vi "Lockin.vi"(4 "stop?":bool, 6 "initialize?":bool, 8 "error in (no error)":errorcluster, 11 "Transport":refnum<class "Transport.lvclass">) -> (0 "error out":errorcluster, 3 "Transport out":refnum<class "Transport.lvclass">)   [LabVIEW 2016, in "Transport.lvclass"]
uses:
  Transport.lvclass
  Control Experiment/Typedefs/Instruments--cluster.ctl
  <userlib>/LevyLab/Krohn Hite 7008/Instrument.KH7008.lvclass
  <userlib>/LevyLab/Lockin-Multichannel/Instrument.Lockin/Instrument.Lockin.lvclass
  <userlib>/LevyLab/Levylab Instruments/Instrument Types/Cryostat/Instrument.Cryostat.lvclass
  <userlib>/LevyLab/Levylab Instruments/Instrument Types/CBridge/Instrument.CBridge.lvclass
  <userlib>/LevyLab/Levylab Instruments/Instrument Types/Optical Delay Line/Instrument.OpticalDelayLine.lvclass
  <userlib>/LevyLab/Levylab Instruments/Instrument Types/Strain/Instrument.Strain.lvclass
  <userlib>/LevyLab/Levylab Instruments/Instrument Types/VNA/Instrument.VNA.lvclass
  <userlib>/LevyLab/Levylab Instruments/Instrument Types/VSource/Instrument.VSource.lvclass
  Transport.lvclass/Transport.ctl
  Control Experiment/Control Experiment.lvclass/Control Experiment.ctl
  SweepControl/SweepControl.lvclass/SweepControl.ctl
  Control Experiment/Control Experiment.lvclass
  SweepControl/SweepControl.lvclass
panel:
  in  "Tab Control":enum32{"lockin/SG Control", "Data", "Other"}(tab)
  out "elapsed time (s)":u32=76
  in  "Experiment Comments":string="describe only the experiment you're doing right now"
  in  "Experiment Folder":string="Experiment folder"
  out "T (mK)":dbl
  out "Field (T)":dbl=0.5 format="%#_13g"
  out "time b/w points (ms)":u32=76
  in  "stop":bool
  out "X Lockins":cluster{dbl[], dbl[]}[](graph)
  out "Y Lockins":cluster{dbl[], dbl[]}[](graph)
  out "G4T":cluster{dbl[], dbl[]}[](graph)
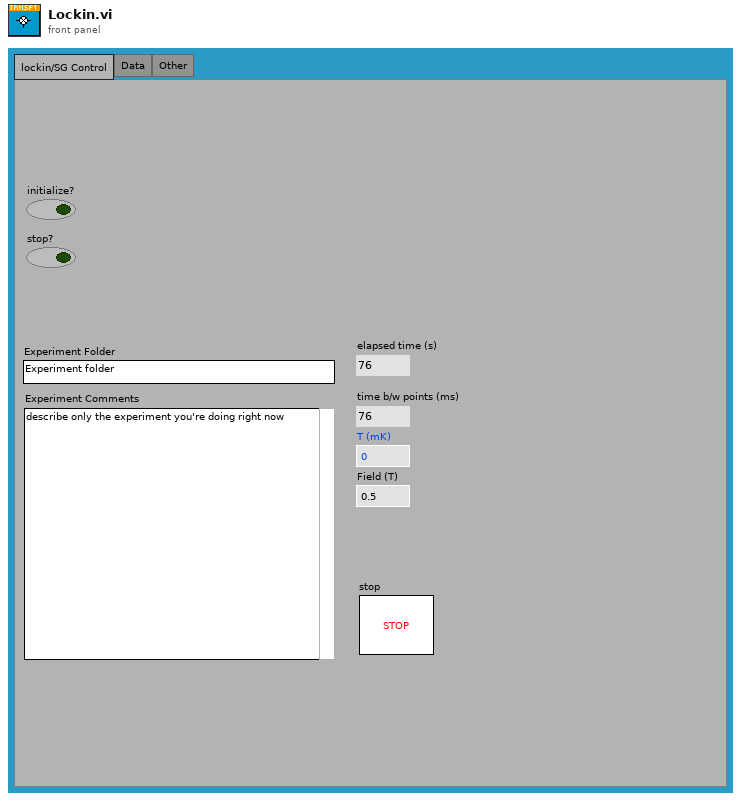
[diagram p1: front panel]
types:
  T1 = enum32{"Invalid", "Standard", "Closed", "Hidden", "Minimized", "Maximized"}
  T2 = enum32{"invalid app kind", "Development System", "Run Time System", "Student Edition", "Embedded LabVIEW", "Evaluation", "Custom"}
  T3 = typedef "Control Experiment.lvclass/Instruments--cluster.ctl" = cluster{"KH7008":refnum<class "Instrument.KH7008.lvclass">[], "Lockin":refnum<class "Instrument.Lockin.lvclass">, "Temperature":refnum<class "Instrument.Cryostat.lvclass">, "Magnet":refnum<class "Instrument.Cryostat.lvclass">, "Rotator":refnum<class "Instrument.Cryostat.lvclass">, "Level":refnum<class "Instrument.Cryostat.lvclass">, "Capacitance Bridge":refnum<class "Instrument.CBridge.lvclass">, "Optical Delay Line":refnum<class "Instrument.OpticalDelayLine.lvclass">, "Strain Cell":refnum<class "Instrument.Strain.lvclass">, "VNA":refnum<class "Instrument.VNA.lvclass">, "Voltage Source":refnum<class "Instrument.VSource.lvclass">}
  T4 = cluster{"Core":cluster{"Current VI Reference":refnum<vi>, "Close Panel on Exit?":bool}, "Transport":refnum<class "Transport.lvclass">, "SweepControl":refnum<class "SweepControl.lvclass">, "Control Experiment":refnum<class "Control Experiment.lvclass">, "Instruments":T3, "Results":dbl[][], "ms [0]":u32, "ms [i]":u32}
  T5 = cluster{"Current VI Reference":refnum<vi>, "Close Panel on Exit?":bool}
  T6 = enum32{"Bad", "Idle", "Run top level", "Running"}
  T7 = cluster{"I-":i32, "I+":i32, "V1-":i32, "V1+":i32, "I2-":i32, "I2+":i32, "V2-":i32, "V2+":i32}
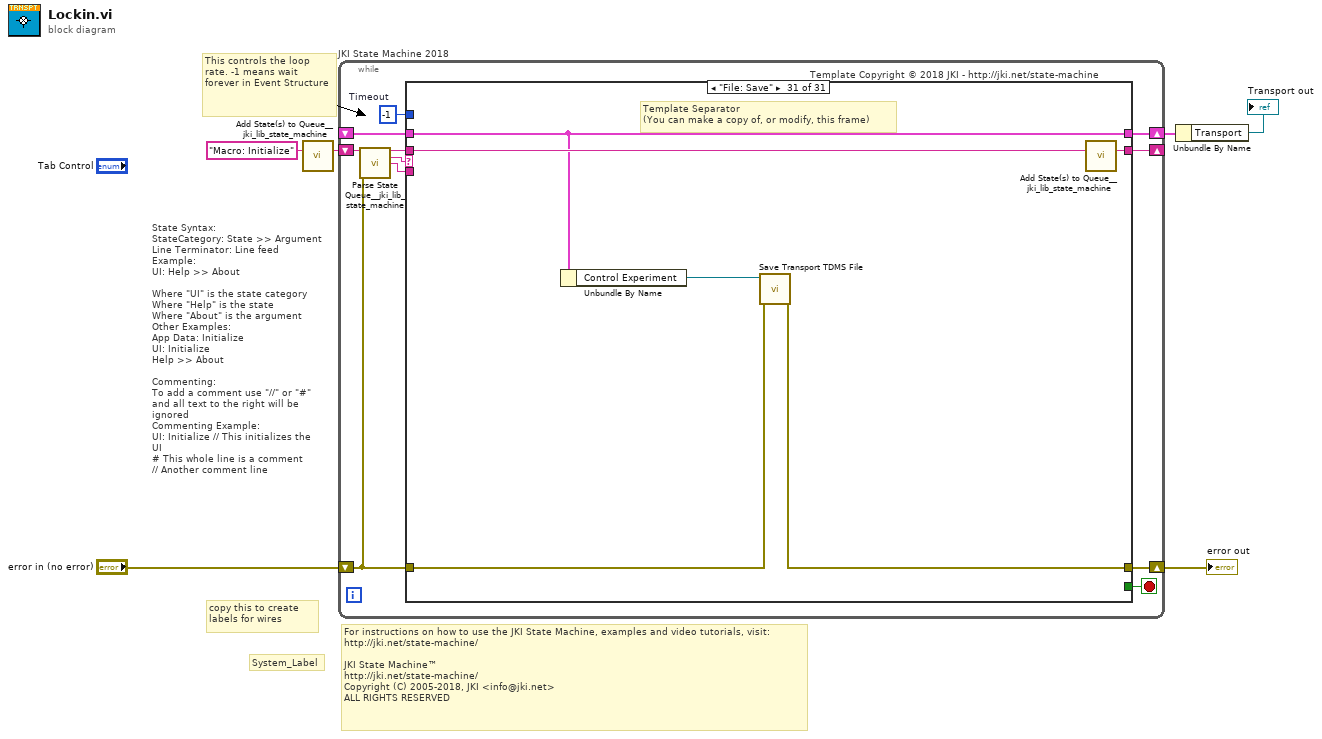
[diagram p0: block diagram]
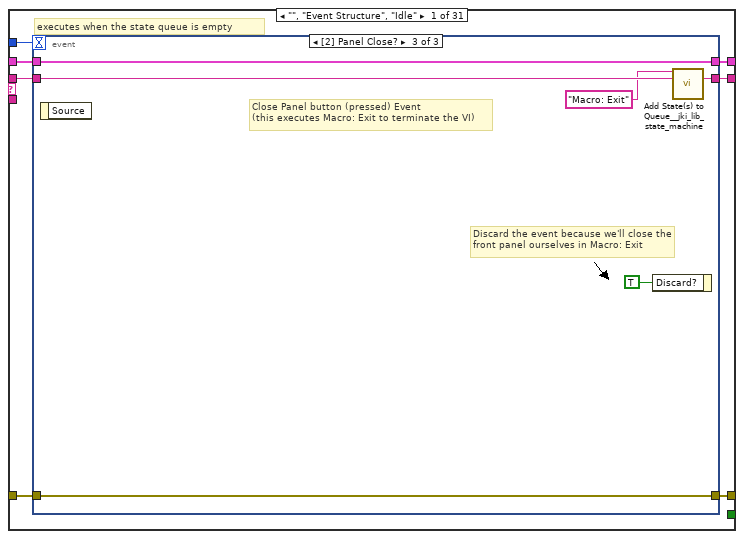
[diagram p2: hidden frame]
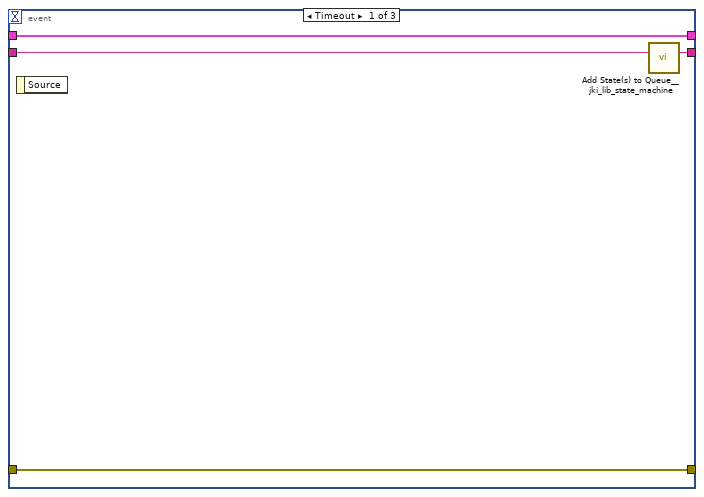
[diagram p3: hidden frame]
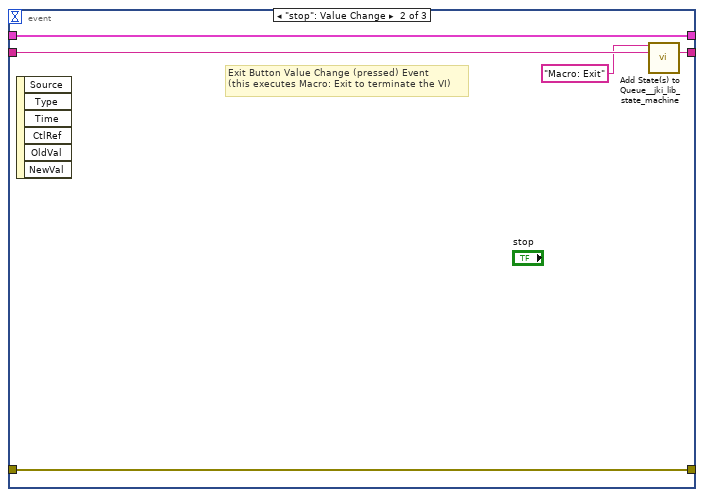
[diagram p4: hidden frame]
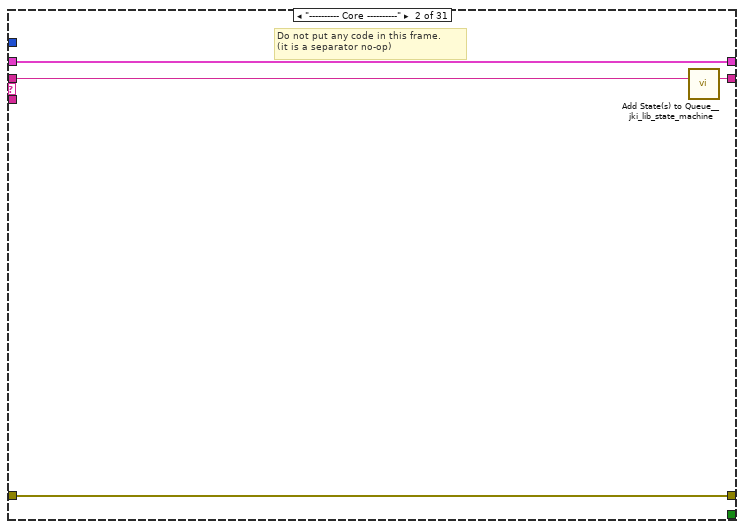
[diagram p5: hidden frame]
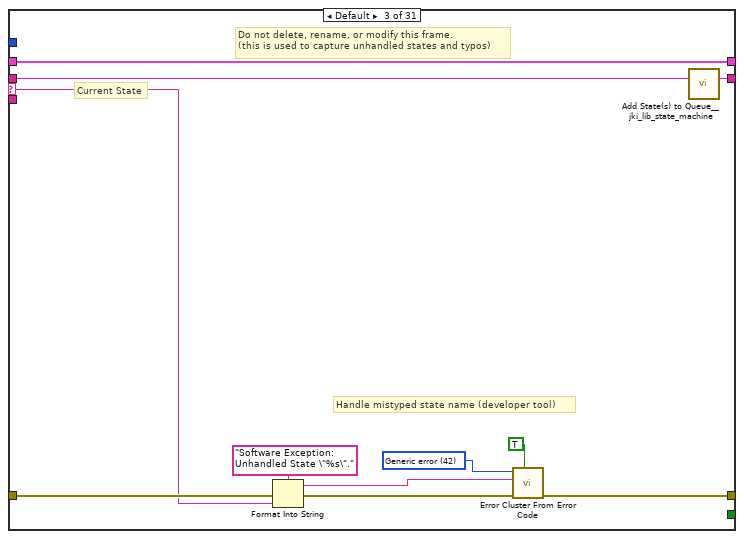
[diagram p6: hidden frame]
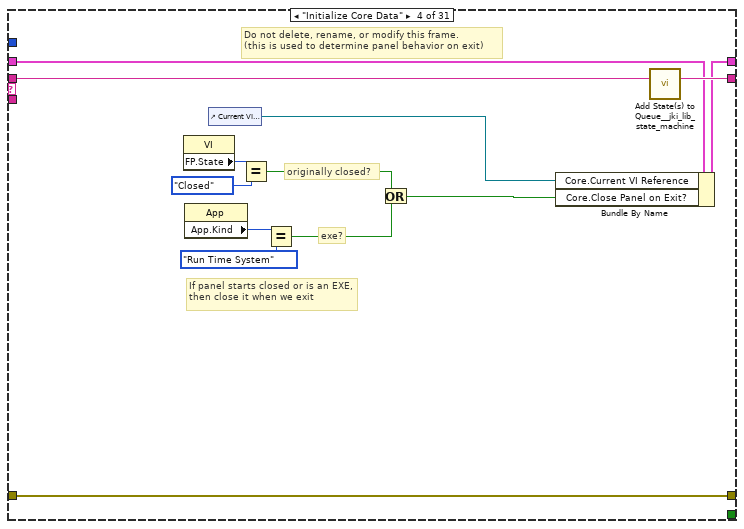
[diagram p7: hidden frame]
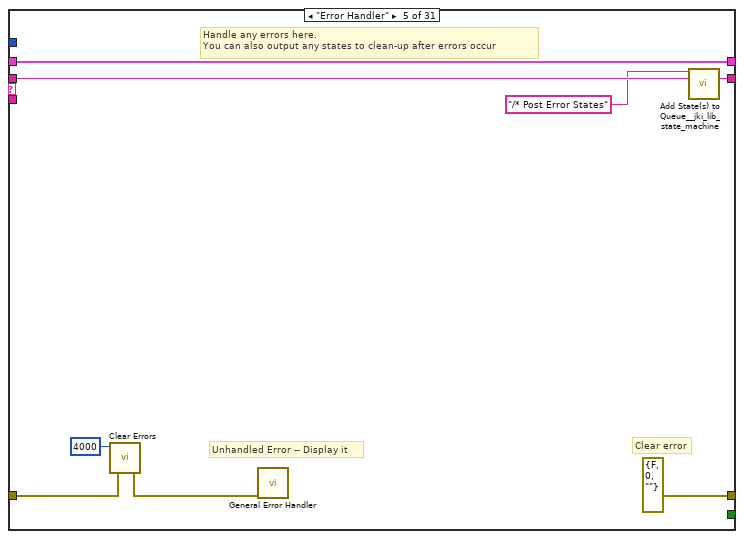
[diagram p8: hidden frame]
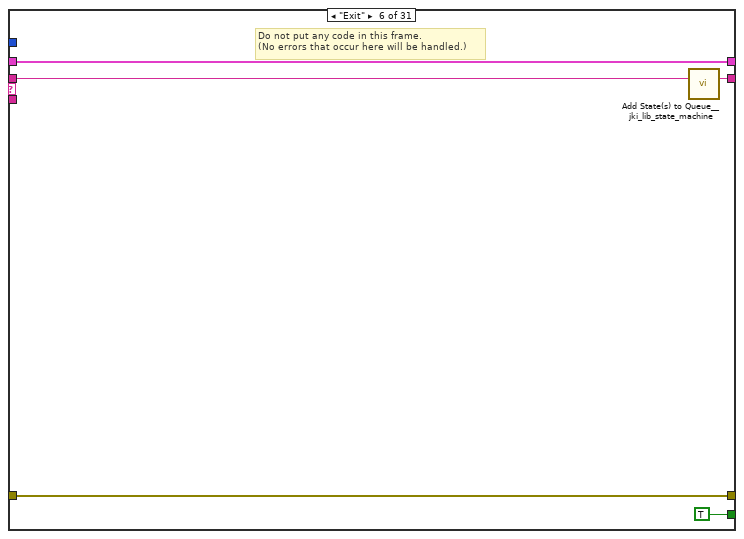
[diagram p9: hidden frame]
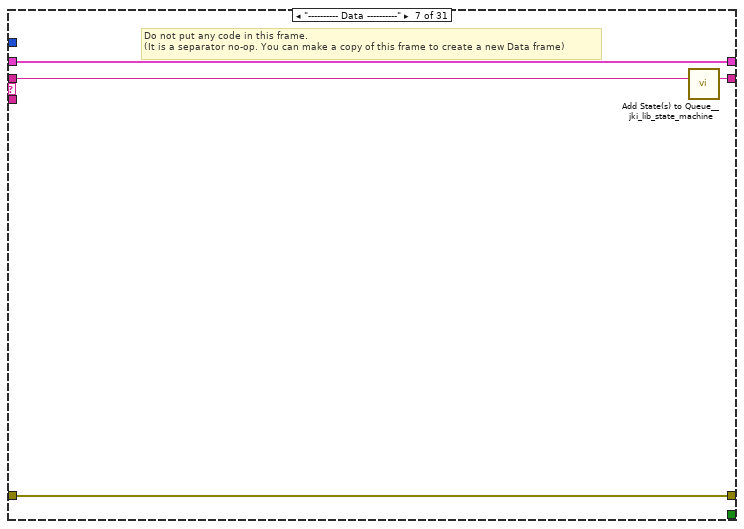
[diagram p10: hidden frame]
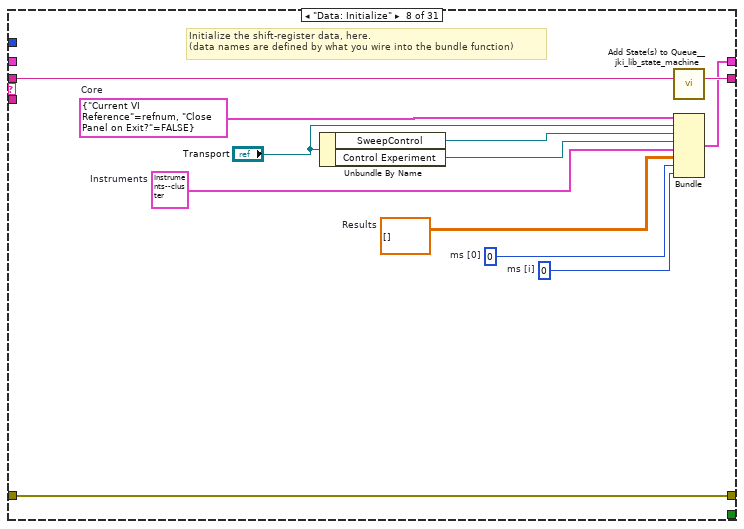
[diagram p11: hidden frame]
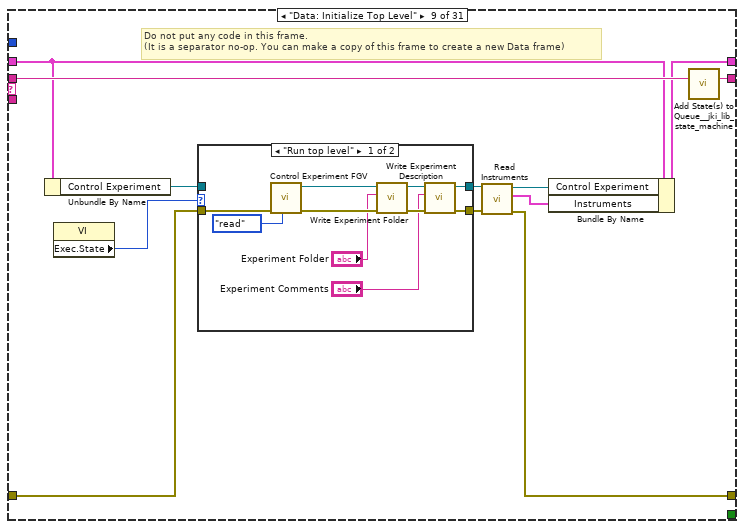
[diagram p12: hidden frame]
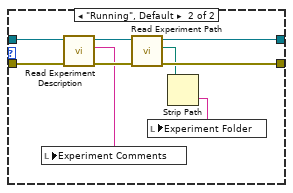
[diagram p13: hidden frame]
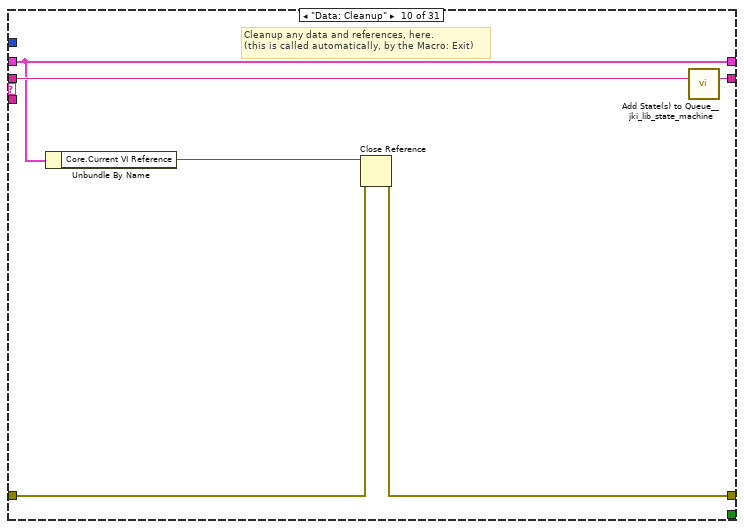
[diagram p14: hidden frame]
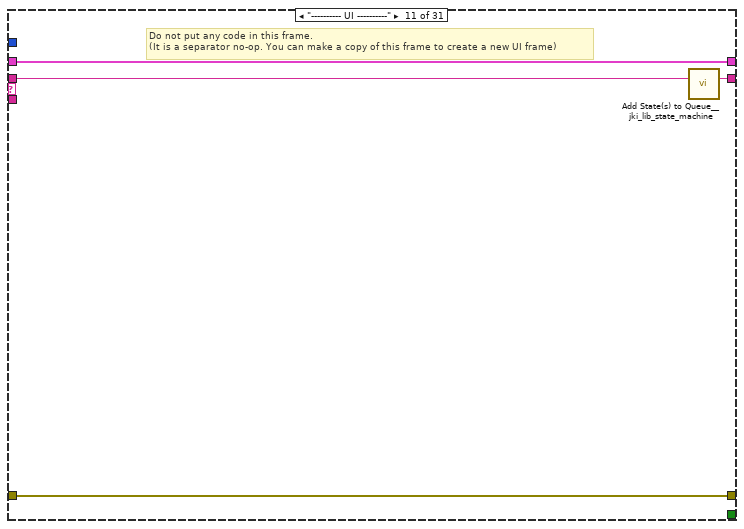
[diagram p15: hidden frame]
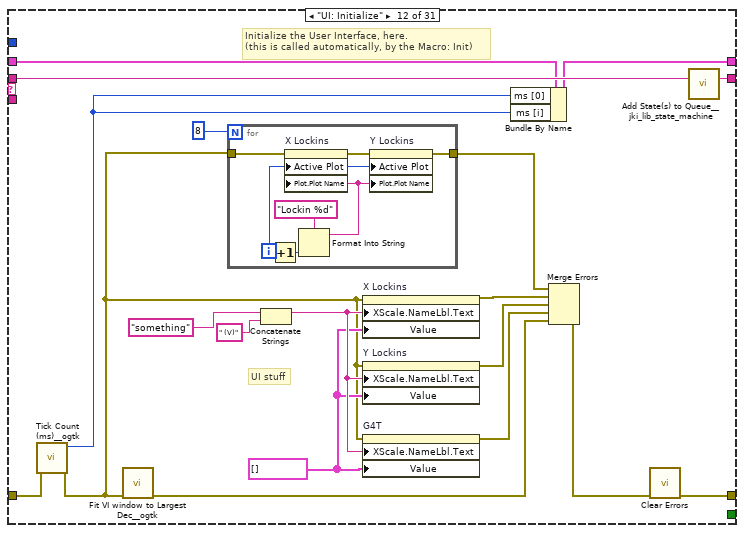
[diagram p16: hidden frame]
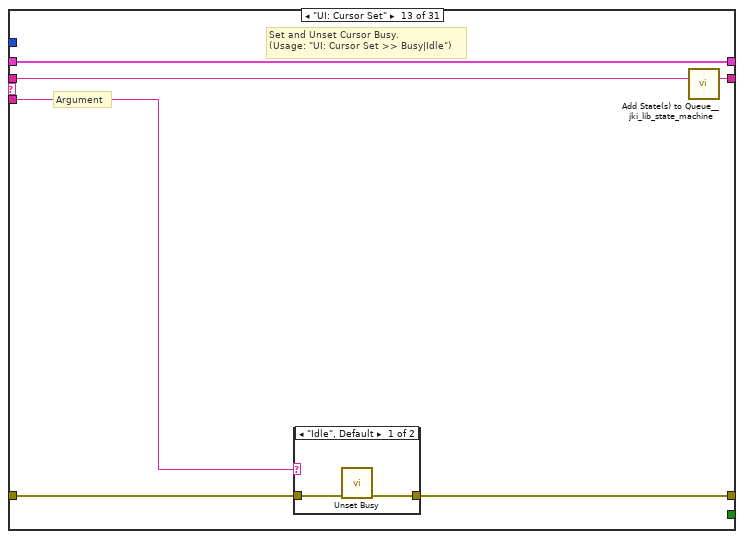
[diagram p17: hidden frame]
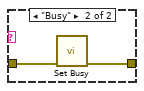
[diagram p18: hidden frame]
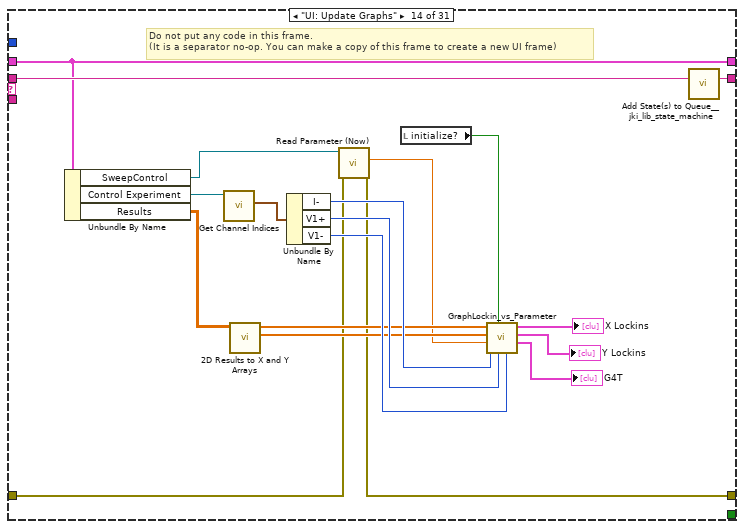
[diagram p19: hidden frame]
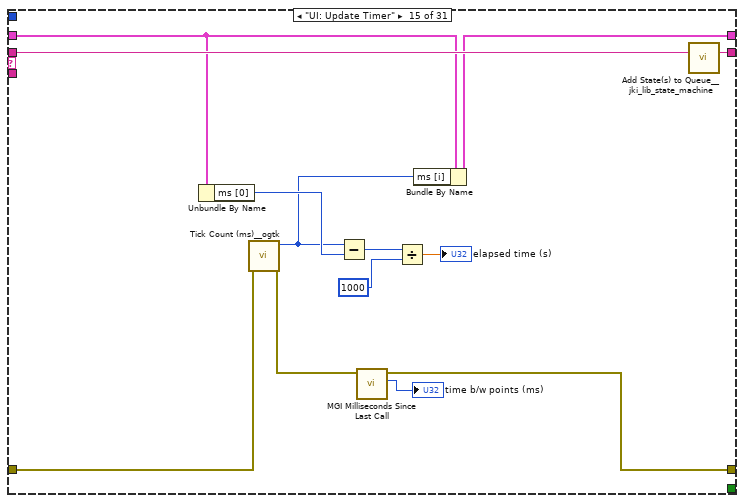
[diagram p20: hidden frame]
diagram:
  # "For instructions on how to use the JKI State Machine, examples and video tutorials, visit:\nhttp://jki.net/state-machine/\n\nJKI State Machine™\nhttp://jki.net/state-machine/\nCopyright (C) 2005-2018, JKI <info@jki.net>\nALL RIGHTS RESERVED"
  # "State Syntax:\nStateCategory: State >> Argument\nLine Terminator: Line feed\nExample:\nUI: Help >> About\n\nWhere \"UI\" is the state category\nWhere \"Help\" is the state\nWhere \"About\" is the argument\nOther Examples:\nApp Data: Initialize\nUI: Initialize\nHelp >> About\n\nCommenting:\nTo add a comment use \"//\" or \"#\" and all text to the right will be ignored\nCommenting Example:\nUI: Initialize // This initializes the UI\n# This whole line is a comment\n// Another comment line"
  # "copy this to create labels for wires"
  # "This controls the loop rate. -1 means wait forever in Event Structure"
  # "System_Label"
  n1 = call <vilib>:"Add State(s) to Queue__jki_lib_state_machine.vi"("State(s) in (\"\")"="Macro: Initialize") -> ("States Out"=w6:string)  [unwired: 14 in]
  n2 = while "JKI State Machine 2018" {
    shift-right: [w10] -> w4
    shift-left: _ -> [w9]
    shift-right: [w13] -> w2
    shift-left: "error in (no error)" -> [w7]
    shift-right: [w12] -> _
    shift-left: w6 -> [w14]
    stop <- w11 stop-if-true
    w8 = -1  # Timeout
    # "Template Copyright © 2018 JKI - http://jki.net/state-machine"
    n3 = call <vilib>:"Parse State Queue__jki_lib_state_machine.vi"("State Queue"=w14, "Error In (no error)"=w7) -> ("Remaining States"=w16:string, "Current State"=w17:string, "Arguments"=w15:string)  [unwired: 11 in]
    n4 = case shown="\"File: Save\"" w17 {
      selector: w17 -> [_ _ w44 _ _ _ _ _ _ _ _ _ _ _ _ _ _ _ _ _ _ _ _ _ _ _ _ _ _ _ _]
      tunnel: w16 -> [w24 w43 w48 w67 w75 w80 w84 w96 w108 w133 w137 w156 w169 w192 w205 w212 w281 w288 w302 w312 w316 w320 w324 w336 w348 w360 w373 w400 w404 w408 w414]
      tunnel: w15 -> [_ _ _ _ _ _ _ _ _ _ _ _ w164 _ _ w206 _ _ _ _ _ _ _ _ _ _ _ _ _ _ _]
      tunnel: w9 -> [w22 w40 w46 w60 w72 w78 w81 _ w98 w128 w134 w143 w167 w179 w200 w208 w278 w286 w299 w309 w313 w317 w321 w332 w345 w349 w368 w396 w401 w405 w412]
      tunnel: [w21 w41 w50 w64 errorcluster {"status"=FALSE, "code"=0, "source"=""} ("error out") w77 w82 w93 w99 w129 w135 w147 w165 w175 w194 w209 w279 w285 w300 w310 w314 w318 w322 w328 w337 w351 w362 w391 w402 w406 w409] -> w13
      tunnel: w7 -> [w20 w41 w49 w64 w69 w77 w82 w93 w100 w130 w135 w144 w166 w176 w202 w210 w279 w285 w300 w310 w314 w318 w322 w333 w342 w352 w371 w392 w402 w406 w410]
      tunnel: [w23 w42 w47 w66 w74 w79 w83 w95 w107 w132 w136 w155 w168 w191 w204 w211 w280 w287 w301 w311 w315 w319 w323 w335 w347 w359 w372 w399 w403 w407 w413] -> w12
      tunnel: [_ _ _ _ _ TRUE _ _ _ _ _ _ _ _ _ _ _ _ _ _ _ _ _ _ _ _ _ _ _ _ _] -> w11
      tunnel: [w19 w40 w46 w65 w72 w78 w81 w94 w97 w128 w134 w142 w167 w179 w199 w208 w278 w286 w299 w309 w313 w317 w321 w331 w344 w354 w369 w397 w401 w405 w412] -> w10
      tunnel: w8 -> [w18 _ _ _ _ _ _ _ _ _ _ _ _ _ _ _ _ _ _ _ _ _ _ _ _ _ _ _ _ _ _]
      frame "", "Event Structure", "Idle" {
        # "executes when the state queue is empty"
        n5 = event shown="[2] Panel Close?" {
          selector: _ -> [_ _ _]
          dyn-events: _ -> [_ _ _]
          timeout: w18 -> [_ _ _]
          tunnel: w24 -> [w28 w33 w39]
          tunnel: [w27 w32 w38] -> w23
          tunnel: w22 -> [w25 w30 w36]
          tunnel: [w26 w31 w37] -> w21
          tunnel: w20 -> [w26 w31 w37]
          tunnel: [w25 w30 w36] -> w19
          event Timeout {
            n6 = event-data() -> ()  [unwired: 1 in, 1 out]
            n7 = call <vilib>:"Add State(s) to Queue__jki_lib_state_machine.vi"("State(s) in (\"\")"=w28) -> ("States Out"=w27:string)  [unwired: 14 in]
          }
          event "stop": Value Change {
            # "Exit Button Value Change (pressed) Event\n(this executes Macro: Exit to terminate the VI)"
            n8 = event-data() -> ()  [unwired: 1 in, 6 out]
            n9 = call <vilib>:"Add State(s) to Queue__jki_lib_state_machine.vi"("State(s) in Front (\"\")"="Macro: Exit", "State(s) in (\"\")"=w33) -> ("States Out"=w32:string)  [unwired: 13 in]
          }
          event Panel Close? {
            # "Discard the event because we'll close the front panel ourselves in Macro: Exit"
            # "Close Panel button (pressed) Event\n(this executes Macro: Exit to terminate the VI)"
            n10 = event-data() -> ()  [unwired: 1 in, 1 out]
            n11 = event-data("Discard?"=TRUE) -> ()  [unwired: 1 in, 1 out]
            n12 = call <vilib>:"Add State(s) to Queue__jki_lib_state_machine.vi"("State(s) in Front (\"\")"="Macro: Exit", "State(s) in (\"\")"=w39) -> ("States Out"=w38:string)  [unwired: 13 in]
          }
        }
      }
      frame "---------- Core ----------" {
        # "Do not put any code in this frame.\n(it is a separator no-op)"
        n13 = call <vilib>:"Add State(s) to Queue__jki_lib_state_machine.vi"("State(s) in (\"\")"=w43) -> ("States Out"=w42:string)  [unwired: 14 in]
      }
      frame Default {
        w53 = 42 items=["No error", "Argument error", "Memory is full", "Out of zone", "End of file", "File already open", "Generic file I/O error", "File not found", "File permission error", "Disk is full", "Duplicate path", "Too many files open", "System feature not enabled", "Resource file not found", "Cannot add resource", "Resource not found", "Image not found", "Image memory error", "Pen does not exist", "Config type invalid", "Config token not found", "Config parse error", "Config memory error", "Bad external code format", "Bad external code offset", "External code not present", "Null window", "Destroy window error", "Null menu", "Print aborted", "Bad print record", "Print driver error", "Windows error during printing", "Memory error during printing", "Print dialog error", "Generic print error", "Invalid device refnum", "Device not found", "Device parameter error", "Device unit error", "Cannot open device", "Device call aborted", "Generic error", "Cancelled by user", "Object ID too low", "Object ID too high", "Object not in heap", "Unknown heap", "Unknown object (invalid DefProc)", "Unknown object (DefProc not in table)", "Message out of range", "Invalid (null) method", "Unknown message", "Manager call not supported", "Bad address", "Network operation in progress", "Network operation timed out", "Connection is busy", "Network attribute not supported", "Network error", "Address in use", "System out of memory", "Connection aborted", "Connection refused", "Not connected", "Already connected", "Connection closed", "Initialization error (interapplication manager)", "Bad occurrence", "Wait on unbound occurrence handler", "Occurrence queue overflow", "Datalog type conflict", "Unused", "Unrecognized type (interapplication manager)", "Memory corrupt", "Failed to make temporary DLL", "Old CIN version", "Drag socket not found", "Failed to load drop-object", "Failed to register OLE object", "Failed to release OLE object", "Format specifier type mismatch", "Unknown format specifier", "Too few format specifiers", "Too many format specifiers", "Scan failed", "Newer CIN version", "Error converting to variant", "Runtime menu error", "Password tampered", "Variant attribute not found", "Incompatible variant data type", "Event data is not available", "Event Store is not present", "Occurrence is not found", "Event Queue is not created", "Event info is not available", "Refnum passed is NULL", "Error retrieving Class GUID", "Error retrieving CoClass GUID", "Error retrieving TypeLib GUID.", "Bad built application magic bytes.", "Specific driver is different from the specific driver associated with the Logical Name.", "There is no session opened to the class driver.", "Max Error", "MAX - Error with config objects", "MAX - Error loading configuration", "MAX - Group not supported"]
        # "Current State"
        # "Do not delete, rename, or modify this frame.\n(this is used to capture unhandled states and typos)"
        # "Handle mistyped state name (developer tool)"
        n14 = Format Into String(format string="Software Exception: Unhandled State \"%s\"." ("message"), error in=w49, w44) -> (resulting string=w52:string, error out=w51:errorcluster)  [unwired: 1 in]
        n15 = call <vilib>:"Error Cluster From Error Code.vi"("show call chain? (False)"=TRUE, "error in (no error)"=w51, "error message (\"\")"=w52, "error code (0)"=w53) -> ("error out"=w50:errorcluster)  [unwired: 5 in]
        n16 = call <vilib>:"Add State(s) to Queue__jki_lib_state_machine.vi"("State(s) in (\"\")"=w48) -> ("States Out"=w47:string)  [unwired: 14 in]
      }
      frame "Initialize Core Data" {
        # "Do not delete, rename, or modify this frame.\n(this is used to determine panel behavior on exit)"
        # "originally closed?"
        # "exe?"
        # "If panel starts closed or is an EXE, then close it when we exit"
        n17 = property class="VI"() -> ("FP.State"=w57:T1)  [unwired: 2 in, 2 out]
        n18 = property class="App"() -> ("App.Kind"=w63:T2)  [unwired: 2 in, 2 out]
        n19 = control-ref of="Current VI Reference"() -> (w58:refnum<vi>)
        n20 = Equal?(x=w57, y=T1."Closed" ("Front Panel Window:State")) -> (x = y?=w55:bool)
        n21 = Equal?(x=w63, y=T2."Run Time System" ("Application:Kind")) -> (x = y?=w61:bool)
        n22 = Or(x=w55, y=w61) -> (x .or. y?=w59:bool)
        n23 = Bundle By Name(cluster=w60, "Core.Current VI Reference"=w58, "Core.Close Panel on Exit?"=w59) -> (w65:T4)
        n24 = call <vilib>:"Add State(s) to Queue__jki_lib_state_machine.vi"("State(s) in (\"\")"=w67) -> ("States Out"=w66:string)  [unwired: 14 in]
      }
      frame "Error Handler" {
        # "Unhandled Error -- Display it"
        # "Handle any errors here.\nYou can also output any states to clean-up after errors occur"
        # "Clear error"
        n25 = call <vilib>:"Clear Errors.vi"("error in (no error)"=w69, "specific error code to clear (0: all)"=4000) -> ("error out"=w68:errorcluster)  [unwired: 4 in, 1 out]
        n26 = call <vilib>:"General Error Handler.vi"("error in (no error)"=w68) -> ()  [unwired: 10 in, 5 out]
        n27 = call <vilib>:"Add State(s) to Queue__jki_lib_state_machine.vi"("State(s) in Front (\"\")"="/* Post Error States", "State(s) in (\"\")"=w75) -> ("States Out"=w74:string)  [unwired: 13 in]
      }
      frame "Exit" {
        # "Do not put any code in this frame.\n(No errors that occur here will be handled.)"
        n28 = call <vilib>:"Add State(s) to Queue__jki_lib_state_machine.vi"("State(s) in (\"\")"=w80) -> ("States Out"=w79:string)  [unwired: 14 in]
      }
      frame "---------- Data ----------" {
        # "Do not put any code in this frame.\n(It is a separator no-op. You can make a copy of this frame to create a new Data frame)"
        n29 = call <vilib>:"Add State(s) to Queue__jki_lib_state_machine.vi"("State(s) in (\"\")"=w84) -> ("States Out"=w83:string)  [unwired: 14 in]
      }
      frame "Data: Initialize" {
        w87 = u32 0  # ms [i]
        w88 = u32 0  # ms [0]
        w89 = dbl[][] []  # Results
        w90 = T3 {"KH7008"=[], "Lockin"=refnum, "Temperature"=refnum, "Magnet"=refnum, "Rotator"=refnum, "Level"=refnum, "Capacitance Bridge"=refnum, "Optical Delay Line"=refnum, "Strain Cell"=refnum, "VNA"=refnum, "Voltage Source"=refnum}  # Instruments
        w92 = T5 {"Current VI Reference"=refnum, "Close Panel on Exit?"=FALSE}  # Core
        # "Initialize the shift-register data, here.\n(data names are defined by what you wire into the bundle function)"
        n30 = Unbundle By Name("Transport") -> ("SweepControl"=w86:refnum<class "SweepControl.lvclass">, "Control Experiment"=w85:refnum<class "Control Experiment.lvclass">)
        n31 = call <vilib>:"Add State(s) to Queue__jki_lib_state_machine.vi"("State(s) in (\"\")"=w96) -> ("States Out"=w95:string)  [unwired: 14 in]
        n32 = Bundle("Core"=w92, "Transport"="Transport", "SweepControl"=w86, "Control Experiment"=w85, "Instruments"=w90, "Results"=w89, "ms [0]"=w88, "ms [i]"=w87) -> (w94:T4)  [unwired: 1 in]
      }
      frame "Data: Initialize Top Level" {
        # "Do not put any code in this frame.\n(It is a separator no-op. You can make a copy of this frame to create a new Data frame)"
        n33 = Unbundle By Name(w98) -> ("Control Experiment"=w101:refnum<class "Control Experiment.lvclass">)
        n34 = property class="VI"() -> ("Exec.State"=w106:T6)  [unwired: 2 in, 2 out]
        n35 = case shown="\"Run top level\"" w106 {
          tunnel: w100 -> [w118 w126]
          tunnel: [w113 w122] -> w102
          tunnel: [w112 w123] -> w103
          tunnel: w101 -> [_ w127]
          frame "Run top level" {
            n36 = call "Control Experiment FGV.vi"("Function"=enum16{"read", "write"}."read", "error in (no error)"=w118) -> ("error out"=w116:errorcluster, "Control Experiment.lvclass out"=w117:refnum<class "Control Experiment.lvclass">)  [unwired: 8 in]
            n37 = call "Write Experiment Folder.vi"("error in (no error)"=w116, "Experiment Folder"="Experiment Folder", "Control Experiment in"=w117) -> ("error out"=w114:errorcluster, "Control Experiment out"=w115:refnum<class "Control Experiment.lvclass">)  [unwired: 7 in]
            n38 = call "Write Experiment Description.vi"("error in (no error)"=w114, "Experiment Description"="Experiment Comments", "Control Experiment in"=w115) -> ("error out"=w113:errorcluster, "Control Experiment out"=w112:refnum<class "Control Experiment.lvclass">)  [unwired: 7 in]
          }
          frame "Running", Default {
            n39 = call "Read Experiment Description.vi"("error in (no error)"=w126, "Control Experiment in"=w127) -> ("error out"=w125:errorcluster, "Experiment Description"=w120:string, "Control Experiment out"=w124:refnum<class "Control Experiment.lvclass">)  [unwired: 7 in]
            n40 = local write "Experiment Comments"(w120) -> ()
            n41 = call "Read Experiment Path.vi"("error in (no error)"=w125, "Control Experiment in"=w124) -> ("error out"=w122:errorcluster, "Experiment Path"=w121:path, "Control Experiment out"=w123:refnum<class "Control Experiment.lvclass">)  [unwired: 7 in]
            n42 = Strip Path(path=w121) -> (name=w119:string)  [unwired: 1 out]
            n43 = local write "Experiment Folder"(w119) -> ()
          }
        }
        n44 = call "Read Instruments.vi"("error in (no error)"=w102, "Control Experiment in"=w103) -> ("error out"=w99:errorcluster, "Instruments"=w105:T3, "Control Experiment out"=w104:refnum<class "Control Experiment.lvclass">)  [unwired: 7 in]
        n45 = Bundle By Name(cluster=w98, "Control Experiment"=w104, "Instruments"=w105) -> (w97:T4)
        n46 = call <vilib>:"Add State(s) to Queue__jki_lib_state_machine.vi"("State(s) in (\"\")"=w108) -> ("States Out"=w107:string)  [unwired: 14 in]
      }
      frame "Data: Cleanup" {
        # "Cleanup any data and references, here.\n(this is called automatically, by the Macro: Exit)"
        n47 = Unbundle By Name(w128) -> ("Core.Current VI Reference"=w131:refnum<vi>)
        n48 = Close Reference(reference=w131, error in (no error)=w130) -> (error out=w129:errorcluster)
        n49 = call <vilib>:"Add State(s) to Queue__jki_lib_state_machine.vi"("State(s) in (\"\")"=w133) -> ("States Out"=w132:string)  [unwired: 14 in]
      }
      frame "---------- UI ----------" {
        # "Do not put any code in this frame.\n(It is a separator no-op. You can make a copy of this frame to create a new UI frame)"
        n50 = call <vilib>:"Add State(s) to Queue__jki_lib_state_machine.vi"("State(s) in (\"\")"=w137) -> ("States Out"=w136:string)  [unwired: 14 in]
      }
      frame "UI: Initialize" {
        w140 = cluster{dbl[], dbl[]}[] [] ("G4T")
        # "UI stuff"
        # "Initialize the User Interface, here.\n(this is called automatically, by the Macro: Init)"
        n51 = call <userlib>:"Tick Count (ms)__ogtk.vi"("error in (no error)"=w144) -> ("error out"=w138:errorcluster, "millisecond timer value"=w141:u32)  [unwired: 9 in]
        n52 = call <userlib>:"Fit VI window to Largest Dec__ogtk.vi"("error in (no error)"=w138) -> ("error out"=w146:errorcluster)  [unwired: 5 in, 1 out]
        n53 = for {
          N: 8 -> [_]
          tunnel: [w157] -> w151
          tunnel: w138 -> [w162]
          i -> [w160]
          n54 = Increment(x=w160) -> (x+1=w158:i32)
          n55 = Format Into String(format string="Lockin %d", w158) -> (resulting string=w161:string)  [unwired: 2 in, 1 out]
          n56 = property on="X Lockins" class="XYGraph (strict)"(error in=w162, "Active Plot"=w160, "Plot.Plot Name"=w161) -> (error out=w159:errorcluster)  [unwired: 1 in, 1 out]
          n57 = property on="Y Lockins" class="XYGraph (strict)"(error in=w159, "Active Plot"=w160, "Plot.Plot Name"=w161) -> (error out=w157:errorcluster)  [unwired: 1 in, 1 out]
        }
        n58 = Concatenate Strings("something" ("string"), " (V)" ("string")) -> (w150:string)
        n59 = property on="X Lockins" class="XYGraph (strict)"(error in=w138, "XScale.NameLbl.Text"=w150, "Value"=w140) -> (error out=w152:errorcluster)  [unwired: 1 in, 1 out]
        n60 = property on="Y Lockins" class="XYGraph (strict)"(error in=w138, "XScale.NameLbl.Text"=w150, "Value"=w140) -> (error out=w153:errorcluster)  [unwired: 1 in, 1 out]
        n61 = property on="G4T" class="XYGraph (strict)"(error in=w138, "XScale.NameLbl.Text"=w150, "Value"=w140) -> (error out=w154:errorcluster)  [unwired: 1 in, 1 out]
        n62 = Bundle By Name(cluster=w143, "ms [0]"=w141, "ms [i]"=w141) -> (w142:T4)
        n63 = Merge Errors(w151, w152, w153, w154, w146) -> (w145:errorcluster)
        n64 = call <vilib>:"Clear Errors.vi"("error in (no error)"=w145) -> ("error out"=w147:errorcluster)  [unwired: 5 in, 1 out]
        n65 = call <vilib>:"Add State(s) to Queue__jki_lib_state_machine.vi"("State(s) in (\"\")"=w156) -> ("States Out"=w155:string)  [unwired: 14 in]
      }
      frame "UI: Cursor Set" {
        # "Argument"
        # "Set and Unset Cursor Busy.\n(Usage: \"UI: Cursor Set >> Busy|Idle\")"
        n66 = case shown="\"Idle\", Default" w164 {
          tunnel: w166 -> [w171 w173]
          tunnel: [w170 w172] -> w165
          frame "Idle", Default {
            n67 = call <vilib>:"Unset Busy.vi"("error in (no error)"=w171) -> ("error out"=w170:errorcluster)  [unwired: 10 in]
          }
          frame "Busy" {
            n68 = call <vilib>:"Set Busy.vi"("error in (no error)"=w173) -> ("error out"=w172:errorcluster)  [unwired: 9 in, 1 out]
          }
        }
        n69 = call <vilib>:"Add State(s) to Queue__jki_lib_state_machine.vi"("State(s) in (\"\")"=w169) -> ("States Out"=w168:string)  [unwired: 14 in]
      }
      frame "UI: Update Graphs" {
        # "Do not put any code in this frame.\n(It is a separator no-op. You can make a copy of this frame to create a new UI frame)"
        n70 = Unbundle By Name(w179) -> ("SweepControl"=w177:refnum<class "SweepControl.lvclass">, "Control Experiment"=w189:refnum<class "Control Experiment.lvclass">, "Results"=w182:dbl[][])
        n71 = call "Get Channel Indices.vi"("Control Experiment in"=w189) -> ("Indices"=w188:T7)  [unwired: 8 in, 2 out]
        n72 = call "2D Results to X and Y Arrays.vi"("Results"=w182) -> ("Y"=w180:dbl[], "X"=w181:dbl[])  [unwired: 9 in]
        n73 = Unbundle By Name(w188) -> ("I-"=w185:i32, "V1+"=w187:i32, "V1-"=w186:i32)
        n74 = call "Read Parameter (Now).vi"("error in (no error)"=w176, "SweepControl in"=w177) -> ("error out"=w175:errorcluster, "Parameter (Now)"=w174:dbl)  [unwired: 7 in, 1 out]
        n75 = local read "initialize?"() -> (w178:bool)
        n76 = call "GraphLockin_vs_Parameter.vi"("V-"=w186, "V+"=w187, "reset?"=w178, "Current"=w185, "Parameter"=w174, "Y[ ]"=w180, "X[ ]"=w181) -> ("G(e2/h) vs Parameter"=→"G4T":cluster{"Y":dbl[], "Y":dbl[]}[], "Y vs Parameter"=→"Y Lockins":cluster{dbl[], dbl[]}[], "X vs Parameter"=→"X Lockins":cluster{dbl[], dbl[]}[])  [unwired: 1 in, 1 out]
        n77 = call <vilib>:"Add State(s) to Queue__jki_lib_state_machine.vi"("State(s) in (\"\")"=w192) -> ("States Out"=w191:string)  [unwired: 14 in]
      }
      frame "UI: Update Timer" {
        n78 = Unbundle By Name(w200) -> ("ms [0]"=w201:u32)
        n79 = call <userlib>:"Tick Count (ms)__ogtk.vi"("error in (no error)"=w202) -> ("error out"=w195:errorcluster, "millisecond timer value"=w193:u32)  [unwired: 9 in]
        n80 = Subtract(x=w193, y=w201) -> (x-y=w197:u32)
        n81 = call <userlib>:"MGI Milliseconds Since Last Call.vi"("Error In"=w195) -> ("ms"=→"time b/w points (ms)":u32, "Error Out"=w194:errorcluster)  [unwired: 5 in]
        n82 = Divide(x=w197, y=u32 1000 ("x")) -> (x/y=→"elapsed time (s)":dbl)
        n83 = Bundle By Name(cluster=w200, "ms [i]"=w193) -> (w199:T4)
        n84 = call <vilib>:"Add State(s) to Queue__jki_lib_state_machine.vi"("State(s) in (\"\")"=w205) -> ("States Out"=w204:string)  [unwired: 14 in]
      }
      frame "UI: Front Panel State" {
        # "Argument"
        # "Set Front Panel Open or Closed\n(Usage: \"UI: Front Panel State >> Open|Close\")"
        n85 = Unbundle By Name(w208) -> ("Core.Current VI Reference"=w207:refnum<vi>)
        n86 = case shown="\"Minimize\", \"Minimized\"" w206 {
          tunnel: w210 -> [w218 w233 w244 w257 w270]
          tunnel: [w220 w234 w246 w259 w272] -> w209
          tunnel: w207 -> [w219 w231 w245 w258 w271]
          frame "Open", "Standard", Default {
            w213 = T1."Standard" ("State")
            n87 = property class="VI"(reference=w219, error in=w218) -> (reference out=w216:refnum<vi>, error out=w217:errorcluster, "FP.State"=w215:T1)
            n88 = Not Equal?(x=w215, y=w213) -> (x != y?=w214:bool)
            n89 = case shown="True" w214 {
              tunnel: [w224 w226] -> w220
              tunnel: w217 -> [w223 w226]
              tunnel: w216 -> [w222 _]
              tunnel: w213 -> [w221 _]
              frame True {
                n90 = invoke class="VI" method="FP.Open"(reference=w222, error in=w223, "Activate"=TRUE, "State"=w221) -> (error out=w224:errorcluster)  [unwired: 1 in, 4 out]
              }
              frame False {
              }
            }
          }
          frame "Close", "Closed" {
            n91 = property class="VI"(reference=w231, error in=w233) -> (reference out=w230:refnum<vi>, error out=w232:errorcluster, "FP.State"=w228:T1)
            n92 = Not Equal?(x=w228, y=T1."Closed" ("Front Panel Window:State")) -> (x != y?=w227:bool)
            n93 = case shown="True" w227 {
              tunnel: [w235 w238] -> w234
              tunnel: w232 -> [w235 w237]
              tunnel: w230 -> [_ w236]
              frame False {
              }
              frame True {
                n94 = invoke class="VI" method="FP.Close"(reference=w236, error in=w237) -> (error out=w238:errorcluster)  [unwired: 1 in, 2 out]
              }
            }
          }
          frame "Hidden", "Hide" {
            w239 = T1."Hidden" ("State")
            n95 = property class="VI"(reference=w245, error in=w244) -> (reference out=w242:refnum<vi>, error out=w243:errorcluster, "FP.State"=w241:T1)
            n96 = Not Equal?(x=w241, y=w239) -> (x != y?=w240:bool)
            n97 = case shown="True" w240 {
              tunnel: [w250 w251] -> w246
              tunnel: w243 -> [w249 w251]
              tunnel: w242 -> [w248 _]
              tunnel: w239 -> [w247 _]
              frame True {
                n98 = invoke class="VI" method="FP.Open"(reference=w248, error in=w249, "State"=w247) -> (error out=w250:errorcluster)  [unwired: 2 in, 4 out]
              }
              frame False {
              }
            }
          }
          frame "Minimize", "Minimized" {
            w252 = T1."Minimized" ("State")
            n99 = property class="VI"(reference=w258, error in=w257) -> (reference out=w255:refnum<vi>, error out=w256:errorcluster, "FP.State"=w254:T1)
            n100 = Not Equal?(x=w254, y=w252) -> (x != y?=w253:bool)
            n101 = case shown="True" w253 {
              tunnel: [w263 w264] -> w259
              tunnel: w256 -> [w262 w264]
              tunnel: w255 -> [w261 _]
              tunnel: w252 -> [w260 _]
              frame True {
                n102 = invoke class="VI" method="FP.Open"(reference=w261, error in=w262, "State"=w260) -> (error out=w263:errorcluster)  [unwired: 2 in, 4 out]
              }
              frame False {
              }
            }
          }
          frame "Maximize", "Maximized" {
            w265 = T1."Maximized" ("State")
            n103 = property class="VI"(reference=w271, error in=w270) -> (reference out=w268:refnum<vi>, error out=w269:errorcluster, "FP.State"=w267:T1)
            n104 = Not Equal?(x=w267, y=w265) -> (x != y?=w266:bool)
            n105 = case shown="True" w266 {
              tunnel: [w276 w277] -> w272
              tunnel: w269 -> [w275 w277]
              tunnel: w268 -> [w274 _]
              tunnel: w265 -> [w273 _]
              frame True {
                n106 = invoke class="VI" method="FP.Open"(reference=w274, error in=w275, "State"=w273) -> (error out=w276:errorcluster)  [unwired: 2 in, 4 out]
              }
              frame False {
              }
            }
          }
        }
        n107 = call <vilib>:"Add State(s) to Queue__jki_lib_state_machine.vi"("State(s) in (\"\")"=w212) -> ("States Out"=w211:string)  [unwired: 14 in]
      }
      frame "---------- Macro ----------" {
        # "Do not put any code in this frame.\n(It is a separator no-op. You can make a copy of this frame to create a new Macro frame)"
        n108 = call <vilib>:"Add State(s) to Queue__jki_lib_state_machine.vi"("State(s) in (\"\")"=w281) -> ("States Out"=w280:string)  [unwired: 14 in]
      }
      frame "Macro: Initialize" {
        w283 = "Data: Initialize\nInitialize Core Data\nUI: Initialize\nUI: Front Panel State >> Open\nData: Initialize Top Level\nMeasure: Temperature\nMeasure: Magnet\nMeasure: Capacitance\nSweep: Initialize\nMacro: Sweep"
        # "Initialization Macro\n(This is called once, when the VI starts)"
        n109 = Select(t=w283, s="initialize?", f="Data: Initialize\nInitialize Core Data\nMacro: Sweep") -> ()  [unwired: 1 out]
        n110 = call <vilib>:"Add State(s) to Queue__jki_lib_state_machine.vi"("State(s) in Front (\"\")"=w283, "State(s) in (\"\")"=w288) -> ("States Out"=w287:string)  [unwired: 13 in]
      }
      frame "Macro: Sweep" {
        # "stop if true"
        n111 = local read "stop"() -> (w294:bool)
        n112 = And(x=w294, y="stop?") -> (x .and. y?=w295:bool)
        n113 = Select(t="File: Save" ("State(s) in Front (\"\")"), s=w295, f="" ("State(s) in Front (\"\")")) -> (s? t:f=w290:string)
        n114 = call <vilib>:"Add State(s) to Queue__jki_lib_state_machine.vi"("State(s) in Front (\"\")"=w290, "State(s) at Back (\"\")"="Macro: Exit" ("State(s) in Front (\"\")")) -> ("States Out"=w289:string)  [unwired: 13 in]
        n115 = call <vilib>:"Add State(s) to Queue__jki_lib_state_machine.vi"("State(s) in Front (\"\")"="Measure: Lockin\nMeasure: Time\n//Measure: Temperature\nUI: Update Graphs\nUI: Update Timer" ("State(s) in Front (\"\")"), "State(s) at Back (\"\")"=w289) -> ("States Out"=w297:string)  [unwired: 13 in]
        n116 = call <vilib>:"Add State(s) to Queue__jki_lib_state_machine.vi"("State(s) in (\"\")"=w302, "State(s) at Back (\"\")"=w297) -> ("States Out"=w301:string)  [unwired: 13 in]
      }
      frame "Macro: Exit" {
        # "Exit Macro\n(This is called once, when the VI exits)"
        n117 = Unbundle By Name(w309) -> ("Core.Close Panel on Exit?"=w308:bool)
        n118 = Select(t="UI: Front Panel State >> Close", s=w308, f="") -> (s? t:f=w305:string)
        n119 = call <vilib>:"Add State(s) to Queue__jki_lib_state_machine.vi"("State(s) in (\"\")"=w305, "State(s) at Back (\"\")"="Data: Cleanup\nExit") -> ("States Out"=w303:string)  [unwired: 13 in]
        n120 = call <vilib>:"Add State(s) to Queue__jki_lib_state_machine.vi"("State(s) in Front (\"\")"=w303, "State(s) in (\"\")"=w312) -> ("States Out"=w311:string)  [unwired: 13 in]
      }
      frame "---------- Sweep ----------" {
        # "Do not put any code in this frame.\n(It is a separator no-op. You can make a copy of this frame to create a new Macro frame)"
        n121 = call <vilib>:"Add State(s) to Queue__jki_lib_state_machine.vi"("State(s) in (\"\")"=w316) -> ("States Out"=w315:string)  [unwired: 14 in]
      }
      frame "---------- Configure ----------" {
        # "Do not put any code in this frame.\n(It is a separator no-op. You can make a copy of this frame to create a new Macro frame)"
        n122 = call <vilib>:"Add State(s) to Queue__jki_lib_state_machine.vi"("State(s) in (\"\")"=w320) -> ("States Out"=w319:string)  [unwired: 14 in]
      }
      frame "---------- Measure ----------" {
        # "Template Separator\n(You can make a copy of, or modify, this frame)"
        n123 = call <vilib>:"Add State(s) to Queue__jki_lib_state_machine.vi"("State(s) in (\"\")"=w324) -> ("States Out"=w323:string)  [unwired: 14 in]
      }
      frame "Measure: Temperature" {
        # "Your code here.\n(You can make a copy of, or modify, this frame)"
        n124 = Unbundle By Name(w332) -> ("Control Experiment"=w327:refnum<class "Control Experiment.lvclass">, "Instruments.Temperature"=w334:refnum<class "Instrument.Cryostat.lvclass">)
        n125 = call-dynamic "Get Temperature.vi"("error in (no error)"=w333, "Instrument.Cryostat in"=w334) -> ("error out"=w329:errorcluster, "Temperature (K)"=w325:dbl)  [unwired: 6 in, 2 out]
        "T (mK)" <- w325
        n126 = call "Write Dictionary Element.vi"("error in (no error)"=w329, "value"=w325, "key"="Temperature", "Control Experiment in"=w327) -> ("error out"=w328:errorcluster, "Control Experiment out"=w326:refnum<class "Control Experiment.lvclass">)  [unwired: 6 in]
        n127 = Bundle By Name(cluster=w332, "Control Experiment"=w326) -> (w331:T4)
        n128 = call <vilib>:"Add State(s) to Queue__jki_lib_state_machine.vi"("State(s) in (\"\")"=w336) -> ("States Out"=w335:string)  [unwired: 14 in]
      }
      frame "Measure: Magnet" {
        # "Your code here.\n(You can make a copy of, or modify, this frame)"
        n129 = Unbundle By Name(w345) -> ("Control Experiment"=w340:refnum<class "Control Experiment.lvclass">, "Instruments.Magnet"=w346:refnum<class "Instrument.Cryostat.lvclass">)
        n130 = call-dynamic "Get Magnet Field.vi"("error in (no error)"=w342, "Instrument.Cryostat in"=w346) -> ("error out"=w343:errorcluster, "B Field (T)"=w339:dbl)  [unwired: 6 in, 2 out]
        "Field (T)" <- w339
        n131 = call "Write Dictionary Element.vi"("error in (no error)"=w343, "value"=w339, "key"="Magnet", "Control Experiment in"=w340) -> ("error out"=w337:errorcluster, "Control Experiment out"=w341:refnum<class "Control Experiment.lvclass">)  [unwired: 6 in]
        n132 = Bundle By Name(cluster=w345, "Control Experiment"=w341) -> (w344:T4)
        n133 = call <vilib>:"Add State(s) to Queue__jki_lib_state_machine.vi"("State(s) in (\"\")"=w348) -> ("States Out"=w347:string)  [unwired: 14 in]
      }
      frame "Measure: Capacitance" {
        # "Your code here.\n(You can make a copy of, or modify, this frame)"
        n134 = Unbundle By Name(w349) -> ("Control Experiment"=w355:refnum<class "Control Experiment.lvclass">, "Instruments.Capacitance Bridge"=w358:refnum<class "Instrument.CBridge.lvclass">)
        n135 = call-dynamic "Get Capacitance.vi"("error in (no error)"=w352, "Instrument.CBridge in"=w358) -> ("error out"=w356:errorcluster, "Capacitance (pF)"=w357:dbl)  [unwired: 7 in, 1 out]
        n136 = call "Write Dictionary Element.vi"("error in (no error)"=w356, "value"=w357, "key"="Capacitance", "Control Experiment in"=w355) -> ("error out"=w351:errorcluster, "Control Experiment out"=w353:refnum<class "Control Experiment.lvclass">)  [unwired: 6 in]
        n137 = Bundle By Name(cluster=w349, "Control Experiment"=w353) -> (w354:T4)
        n138 = call <vilib>:"Add State(s) to Queue__jki_lib_state_machine.vi"("State(s) in (\"\")"=w360) -> ("States Out"=w359:string)  [unwired: 14 in]
      }
      frame "Measure: Lockin" {
        n139 = Unbundle By Name(w368) -> ("Control Experiment"=w364:refnum<class "Control Experiment.lvclass">, "Instruments.Lockin"=w370:refnum<class "Instrument.Lockin.lvclass">)
        n140 = call <userlib>:"waitForNewResults.vi"("error in (no error)"=w371, "Instrument.Lockin in"=w370) -> ("error out"=w363:errorcluster, "Results"=w367:dbl[][])  [unwired: 7 in, 1 out]
        n141 = call "2D Results to X and Y Arrays.vi"("Results"=w367) -> ("Y"=w365:dbl[], "X"=w366:dbl[])  [unwired: 9 in]
        n142 = for {
          tunnel: w366 -> [w383] mode=indexing
          tunnel: w365 -> [w377] mode=indexing
          tunnel: w363 -> [w376]
          tunnel: [w375] -> w362
          shift-right: [w374] -> w361
          shift-left: w364 -> [w386]
          i -> [w389]
          n143 = Increment(x=w389) -> (x+1=w381:i32)
          n144 = Format Into String(format string="X%d" ("wavenames"), error in=w376, w381) -> (resulting string=w385:string, error out=w380:errorcluster)  [unwired: 1 in]
          n145 = call "Append Dictionary Element.vi"("error in (no error)"=w380, "value"=w383, "key"=w385, "Control Experiment in"=w386) -> ("error out"=w379:errorcluster, "Control Experiment out"=w382:refnum<class "Control Experiment.lvclass">)  [unwired: 6 in]
          n146 = Format Into String(format string="Y%d" ("wavenames"), error in=w379, w381) -> (resulting string=w384:string, error out=w378:errorcluster)  [unwired: 1 in]
          n147 = call "Append Dictionary Element.vi"("error in (no error)"=w378, "value"=w377, "key"=w384, "Control Experiment in"=w382) -> ("error out"=w375:errorcluster, "Control Experiment out"=w374:refnum<class "Control Experiment.lvclass">)  [unwired: 6 in]
        }
        n148 = Bundle By Name(cluster=w368, "Results"=w367, "Control Experiment"=w361) -> (w369:T4)
        n149 = call <vilib>:"Add State(s) to Queue__jki_lib_state_machine.vi"("State(s) in (\"\")"=w373) -> ("States Out"=w372:string)  [unwired: 14 in]
      }
      frame "Measure: Time" {
        # "Your code here.\n(You can make a copy of, or modify, this frame)"
        n150 = Unbundle By Name(w396) -> ("Control Experiment"=w395:refnum<class "Control Experiment.lvclass">)
        n151 = Get Date/Time In Seconds() -> (seconds since 1Jan1904=w398:timestamp)
        n152 = To Double Precision Float(number=w398) -> (double precision float=w394:dbl)
        n153 = call "Write Dictionary Element.vi"("error in (no error)"=w392, "value"=w394, "key"="Time", "Control Experiment in"=w395) -> ("error out"=w391:errorcluster, "Control Experiment out"=w390:refnum<class "Control Experiment.lvclass">)  [unwired: 6 in]
        n154 = Bundle By Name(cluster=w396, "Control Experiment"=w390) -> (w397:T4)
        n155 = call <vilib>:"Add State(s) to Queue__jki_lib_state_machine.vi"("State(s) in (\"\")"=w400) -> ("States Out"=w399:string)  [unwired: 14 in]
      }
      frame "---------- File ----------" {
        # "Template Separator\n(You can make a copy of, or modify, this frame)"
        n156 = call <vilib>:"Add State(s) to Queue__jki_lib_state_machine.vi"("State(s) in (\"\")"=w404) -> ("States Out"=w403:string)  [unwired: 14 in]
      }
      frame "File: Configure" {
        # "Template Separator\n(You can make a copy of, or modify, this frame)"
        n157 = call <vilib>:"Add State(s) to Queue__jki_lib_state_machine.vi"("State(s) in (\"\")"=w408) -> ("States Out"=w407:string)  [unwired: 14 in]
      }
      frame "File: Save" {
        # "Template Separator\n(You can make a copy of, or modify, this frame)"
        n158 = Unbundle By Name(w412) -> ("Control Experiment"=w411:refnum<class "Control Experiment.lvclass">)
        n159 = call "Save Transport TDMS File.vi"("error in (no error)"=w410, "Control Experiment in"=w411) -> ("error out"=w409:errorcluster)  [unwired: 8 in, 1 out]
        n160 = call <vilib>:"Add State(s) to Queue__jki_lib_state_machine.vi"("State(s) in (\"\")"=w414) -> ("States Out"=w413:string)  [unwired: 14 in]
      }
    }
  }
  "error out" <- w2
  n161 = Unbundle By Name(w4) -> ("Transport"=→"Transport out":refnum<class "Transport.lvclass">)
